vi "In_S5F3.vi"(8 "error in (no error)":errorcluster, 11 "S5 Message Class in":refnum<class "S5 Message Class.lvclass">) -> (0 "error out":errorcluster, 1 "OK?":bool, 2 "S5F3":T1, 3 "S5 Message Class out":refnum<class "S5 Message Class.lvclass">)   [LabVIEW 2020, in "SECS Communication.lvlib" / "S5 Message Class.lvclass"]
uses:
  S5 Message Class.lvclass
  D:/Dropbox/SECS/SECS_GEM v1.0.6/Com/SECS Communication/SECS-II Class/SECS-II Class.lvclass
  S5F3.ctl
  SECS-II Class/SECS-II Class.lvclass/SECS-II Class.ctl
  SECS-II Class/Variant To Data_Binary.vi
  SECS-II Class/Variant To Data_U4.vi
  SECS-II Class/SECS-II Class.lvclass
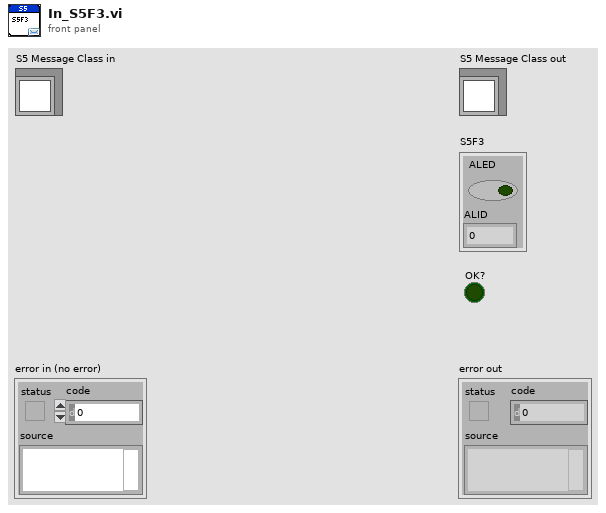
[diagram p1: front panel]
types:
  T1 = typedef "SECS Communication.lvlib/S5 Message Class.lvclass/S5F3.ctl" = cluster{"ALED":bool, "ALID":u32}
  T2 = typedef "SECS Communication.lvlib/SECS-II Class.lvclass/Message Data.ctl" = cluster{"Index":i32, "Data Item Format":T3, "Format Code":T4, "Parent Index":i32, "Child Index":i32[], "Data":variant}
  T3 = typedef "SECS Communication.lvlib/SECS-II Class.lvclass/Data Item Format.ctl" = enum16{"Data Type", "Value"}
  T4 = typedef "SECS Communication.lvlib/SECS-II Class.lvclass/Format Code.ctl" = enum16{"L", "A", "B", "Boolean", "J", "I1", "I2", "I4", "I8", "U1", "U2", "U4", "U8", "F4", "F8", "Char"}
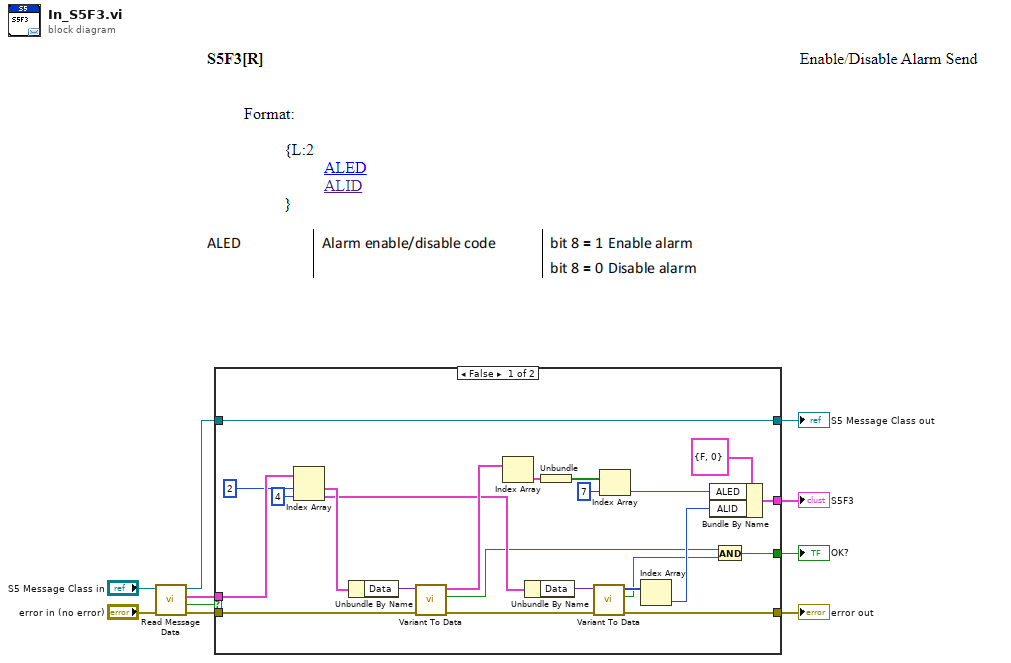
[diagram p0: block diagram]
diagram:
  n1 = call "Read Message Data.vi"("error in (no error)"="error in (no error)", "SECS-II Class in"="S5 Message Class in") -> ("error out"=w9:errorcluster, "Empty?"=w3:bool, "Message Data"=w10:T2[], "SECS-II Class out"=w2:refnum<class "S5 Message Class.lvclass">)  [unwired: 6 in]
  n2 = case shown="False" w3 {
    tunnel: w10 -> [w32 _]
    tunnel: w9 -> [w30 w34]
    tunnel: [w19 _] -> w8
    tunnel: [w18 w34] -> w5
    tunnel: [w15 _] -> w4
    tunnel: w2 -> [w14 w35]
    tunnel: [w14 w35] -> w1
    frame False {
      n3 = Index Array(array=w32, index #1=2 ("index"), index #2=4 ("index")) -> (element #1=w33:T2, element #2=w24:T2)
      n4 = Unbundle By Name(w33) -> ("Data"=w29:variant)
      n5 = call-poly "Variant To Data.vi"("error in (no error)"=w30, "Variant"=w29) -> ("error out"=w26:errorcluster, "OK?"=w16:bool, "Data Cluster"=w27:cluster{"Data":bool[]}[])  [unwired: 7 in]
      n6 = Index Array(array=w27) -> (element=w23:cluster{"Data":bool[]})  [unwired: 1 in]
      n7 = Unbundle By Name(w24) -> ("Data"=w25:variant)
      n8 = Unbundle(w23) -> ("Data"=w13:bool[])
      n9 = call-poly "Variant To Data.vi"("error in (no error)"=w26, "Variant"=w25) -> ("error out"=w18:errorcluster, "OK?"=w17:bool, "Data"=w21:u32[])  [unwired: 7 in]
      n10 = Index Array(array=w13, index=7) -> (element=w11:bool)
      n11 = Index Array(array=w21) -> (element=w20:u32)  [unwired: 1 in]
      n12 = Bundle By Name(cluster=T1 {"ALED"=FALSE, "ALID"=0} ("S5F3"), "ALED"=w11, "ALID"=w20) -> (w19:T1)
      n13 = And(x=w16, y=w17) -> (x .and. y?=w15:bool)
    }
    frame True {
    }
  }
  "error out" <- w5
  "S5 Message Class out" <- w1
  "S5F3" <- w8
  "OK?" <- w4
